vi "SetSerializedData.vi"(0 "reference in":refnum<class "StateDiagramGraph.lvclass">, 2 "SerializedData(XML)":string, 5 "error in (no error)":errorcluster) -> (14 "reference out":refnum<class "StateDiagramGraph.lvclass">, 19 "error out":errorcluster)   [LabVIEW 2016, in "StateDiagramGraph.lvclass"]
uses:
  <resource>/Framework/Providers/Open_GDS/UML/StateDiagramGraph_class/StateDiagramGraph.lvclass
  <resource>/Framework/Providers/Open_GDS/UML/StateDiagramGraph_class/private/StateDiagramData.ctl
  <resource>/Framework/Providers/Open_GDS/UML/StateDiagramGraph_class/private/ViPathShowOption.ctl
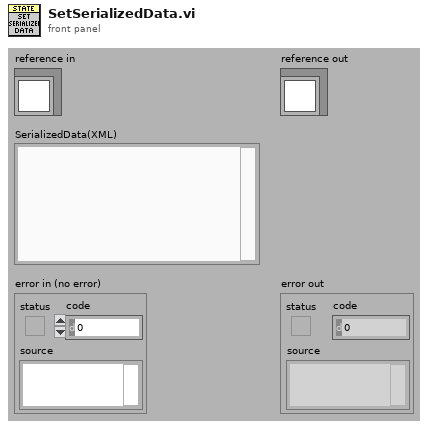
[diagram p1: front panel]
types:
  T1 = typedef "StateDiagramGraph.lvclass/StateDiagramData.ctl" = cluster{"VI-Path":path, "ShowOption":T2}
  T2 = typedef "StateDiagramGraph.lvclass/ViPathShowOption.ctl" = enum16{"Don't Show", "Show Relative Path", "Show Absolute Path"}
  T3 = typedef "StateDiagramGraph.lvclass/ObjectAttributes.ctl" = cluster{"StateDiagramData":T1}
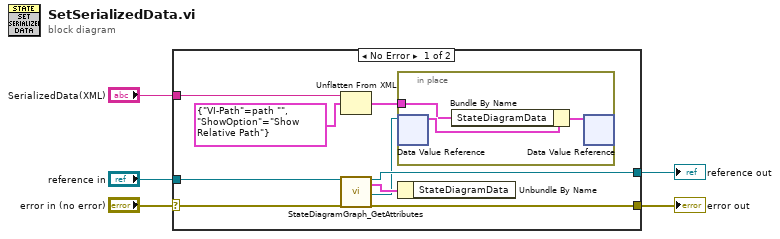
[diagram p0: block diagram]
diagram:
  n1 = case shown="No Error" "error in (no error)" {
    selector: "error in (no error)" -> [w14 w19]
    tunnel: [w12 w19] -> w4
    tunnel: [w10 w18] -> w2
    tunnel: "reference in" -> [w11 w18]
    tunnel: "SerializedData(XML)" -> [w6 _]
    frame No Error {
      n2 = Unflatten From XML(xml string=w6, type=T1 {"VI-Path"=path "", "ShowOption"=enum."Show Relative Path"} ("StateDiagramData")) -> (value=w7:T1)  [unwired: 1 in, 1 out]
      n3 = call <resource>:"StateDiagramGraph_GetAttributes.vi"("reference in"=w11, "error in (no error)"=w14) -> ("reference out"=w10:refnum<class "StateDiagramGraph.lvclass">, "Data"=w13:T3, "DataRef"=w8:refnum<data-value>, "error out"=w12:errorcluster)  [unwired: 14 in]
      n4 = in-place {
        in-place-border: w7 -> [w15]
        n5 = in-place-dvr #1(w8) -> (w17:T3)  [unwired: 1 out]
        n6 = Bundle By Name(cluster=w17, "StateDiagramData"=w15) -> (w16:T3)
        n7 = in-place-dvr #1(w16) -> ()  [unwired: 2 out]
      }
      n8 = Unbundle By Name(w13) -> ()  [unwired: 1 out]
    }
    frame Error {
    }
  }
  "error out" <- w4
  "reference out" <- w2
